vi "GetGXMLCfgFreq.vi"(8 "error in (no error)":errorcluster, 11 "Freq in":refnum<class "Frequency.lvclass">) -> (0 "error out":errorcluster, 2 "FreqChanCfg":T1, 3 "Freq out":refnum<class "Frequency.lvclass">)   [LabVIEW 2018, in "Measurement Channels.lvlib" / "Frequency.lvclass"]
uses:
  Frequency.lvclass
  FreqProps_TD.ctl
  Frequency.lvclass/Frequency.ctl
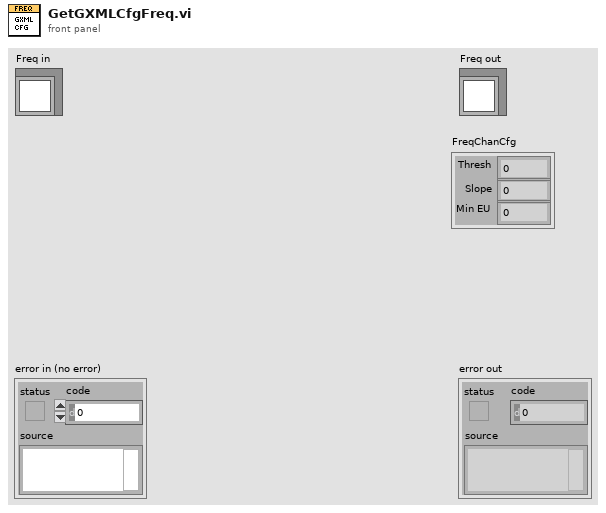
[diagram p1: front panel]
types:
  T1 = typedef "Measurement Channels.lvlib/Frequency.lvclass/FreqProps_TD.ctl" = cluster{"Thresh":dbl, "Slope":u16, "Min EU":dbl}
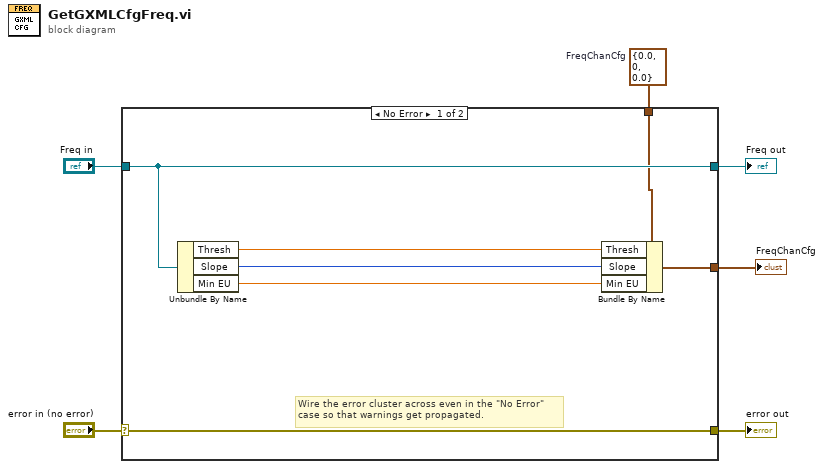
[diagram p0: block diagram]
diagram:
  w2 = T1 {"Thresh"=0.0, "Slope"=0, "Min EU"=0.0}  # FreqChanCfg
  n1 = case shown="No Error" "error in (no error)" {
    selector: "error in (no error)" -> [w13 w16]
    tunnel: [w13 w16] -> w5
    tunnel: [w12 w15] -> w3
    tunnel: "Freq in" -> [w12 w15]
    tunnel: w2 -> [w11 w14]
    tunnel: [w7 w14] -> w1
    frame No Error {
      # "Wire the error cluster across even in the \"No Error\"\ncase so that warnings get propagated."
      n2 = Unbundle By Name(w12) -> ("Thresh"=w10:dbl, "Slope"=w9:u16, "Min EU"=w8:dbl)
      n3 = Bundle By Name(cluster=w11, "Thresh"=w10, "Slope"=w9, "Min EU"=w8) -> (w7:T1)
    }
    frame Error {
    }
  }
  "error out" <- w5
  "Freq out" <- w3
  "FreqChanCfg" <- w1
